vi "Add row to database.vi"(8 "error in (no error)":errorcluster, 11 "Basic Table in":refnum<class "Basic Table.lvclass">) -> (0 "error out":errorcluster, 3 "Basic Table out":refnum<class "Basic Table.lvclass">)   [LabVIEW 2020, in "Table.lvlib" / "Basic Table.lvclass"]
uses:
  Basic Table.lvclass
  Basic Table.lvclass/Basic Table.ctl
  Table Configuration Interface/Table Configuration Interface.lvclass
  Database Libraries/Database Interfaces/Database Interface Class/Database Interface.lvclass
  Column Libraries/Column Interface/Column Interface Class/Column Interface.lvclass
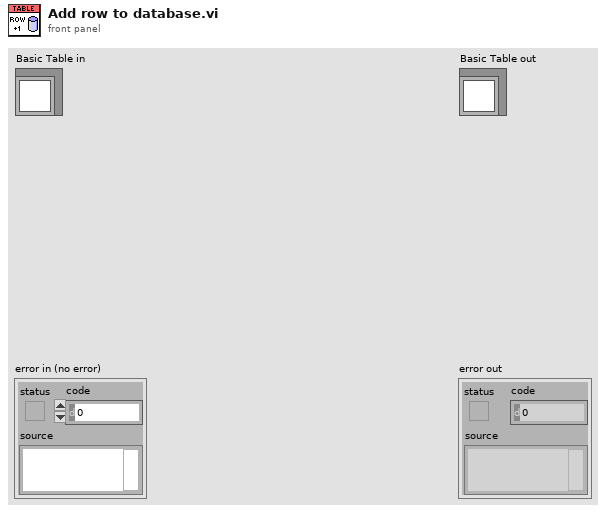
[diagram p1: front panel]
types:
  T1 = map{string, refnum<class "Column Interface.lvclass">}
  T2 = typedef "Database Interfaces.lvlib/Primary Key Info.ctl" = cluster{"Primary Key Column":string, "Display Column":string}
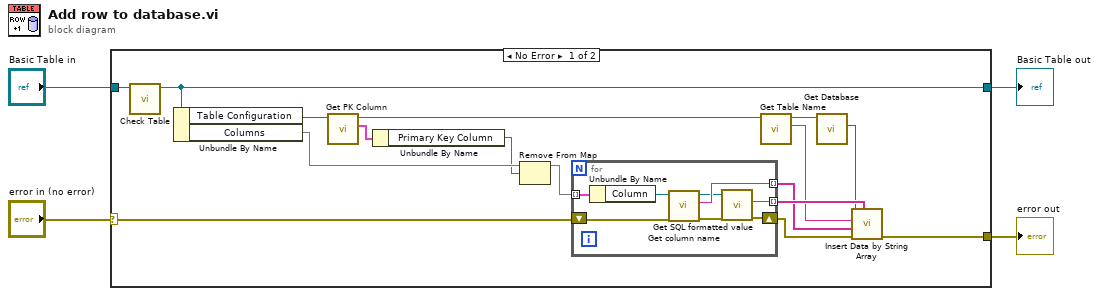
[diagram p0: block diagram]
diagram:
  n1 = case shown="No Error" "error in (no error)" {
    selector: "error in (no error)" -> [w18 w30]
    tunnel: [w12 w30] -> w3
    tunnel: [w19 w29] -> w1
    tunnel: "Basic Table in" -> [w20 w29]
    frame No Error {
      n2 = call "Check Table.vi"("Table in"=w20) -> ("Table out"=w19:refnum<class "Basic Table.lvclass">)  [unwired: 9 in, 1 out]
      n3 = Unbundle By Name(w19) -> ("Table Configuration"=w17:refnum<class "Table Configuration Interface.lvclass">, "Columns"=w14:T1)
      n4 = call-dynamic "Get PK Column.vi"("Table Configuration Interface in"=w17) -> ("Primary Key"=w16:T2, "Table Configuration Interface out"=w5:refnum<class "Table Configuration Interface.lvclass">)  [unwired: 8 in, 1 out]
      n5 = Unbundle By Name(w16) -> ("Primary Key Column"=w13:string)
      n6 = Remove From Map(10:w13, 11:w14) -> (3:w15:T1)  [unwired: 2 out]
      n7 = for {
        tunnel: w15 -> [w28] mode=indexing
        tunnel: [w26] -> w8 mode=indexing
        shift-right: [w23] -> w7
        shift-left: w18 -> [w25]
        tunnel: [w21] -> w11 mode=indexing
        n8 = Unbundle By Name(w28) -> ("Column"=w27:refnum<class "Column Interface.lvclass">)
        n9 = call-dynamic "Get column name.vi"("error in (no error)"=w25, "Column Interface in"=w27) -> ("error out"=w24:errorcluster, "Name"=w26:string, "Column Interface out"=w22:refnum<class "Column Interface.lvclass">)  [unwired: 7 in]
        n10 = call-dynamic "Get SQL formatted value.vi"("error in (no error)"=w24, "Column Interface in"=w22) -> ("error out"=w23:errorcluster, "Formatted Value"=w21:string)  [unwired: 7 in, 1 out]
      }
      n11 = call-dynamic "Get Table Name.vi"("Table Configuration Interface in"=w5) -> ("Table Name"=w9:string, "Table Configuration Interface out"=w6:refnum<class "Table Configuration Interface.lvclass">)  [unwired: 8 in, 1 out]
      n12 = call-dynamic "Get Database.vi"("Table Configuration Interface in"=w6) -> ("Database"=w10:refnum<class "Database Interface.lvclass">)  [unwired: 8 in, 2 out]
      n13 = call-dynamic "Insert Data by String Array.vi"("data"=w11, "error in (no error)"=w7, "columns"=w8, "table"=w9, "Database Interface in"=w10) -> ("error out"=w12:errorcluster)  [unwired: 5 in, 1 out]
    }
    frame Error {
    }
  }
  "error out" <- w3
  "Basic Table out" <- w1
